vi "create or replace existing folder.vi"(8 "error in":errorcluster, 11 "path":path) -> (0 "error out":errorcluster, 3 "created path":path)   [LabVIEW 2014]
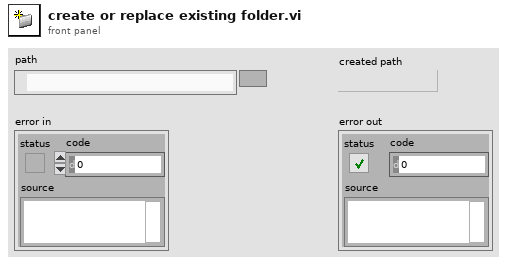
[diagram p1: front panel]
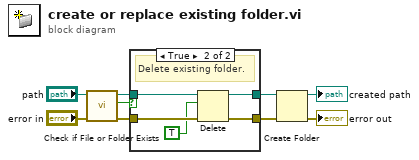
[diagram p0: block diagram]
diagram:
  n1 = call <vilib>:"Check if File or Folder Exists.vi"("error in (no error)"="error in", "path"="path") -> ("error out"=w7:errorcluster, "file or folder exists?"=w5:bool, "dup path"=w6:path)  [unwired: 7 in]
  n2 = case shown="True" w5 {
    tunnel: w6 -> [w11 w15]
    tunnel: w7 -> [w10 w16]
    tunnel: [w11 w13] -> w8
    tunnel: [w10 w12] -> w9
    frame False {
    }
    frame True {
      # "Delete existing folder."
      n3 = Delete(path (use dialog)=w15, entire hierarchy (F)=TRUE, error in=w16) -> (deleted path=w13:path, error out=w12:errorcluster)  [unwired: 2 in, 1 out]
    }
  }
  n4 = Create Folder(path (use dialog)=w8, error in=w9) -> (created path=→"created path":path, error out=→"error out":errorcluster)  [unwired: 1 in, 1 out]
